vi "test - FGV Register and Unregister.vi"(8 "error in (no error)":errorcluster, 11 "TestCase in":refnum<class "testcase-Broadcast Registry.lvclass">) -> (0 "error out":errorcluster, 3 "TestCase out":refnum<class "testcase-Broadcast Registry.lvclass">)   [LabVIEW 2017, in "testcase-Broadcast Registry.lvclass"]
uses:
  testcase-Broadcast Registry.lvclass
  <vilib>/addons/_JKI Toolkits/VI Tester/TestCase.llb/TestCase.lvclass
  C:/Program Files (x86)/National Instruments/LabVIEW 2017/vi.lib/addons/_JKI Toolkits/VI Tester/TestCase.llb/TestCase.lvclass
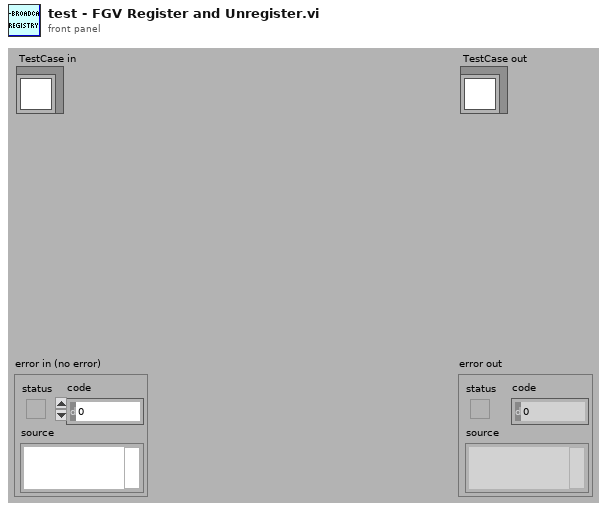
[diagram p1: front panel]
types:
  T1 = cluster{"response message":string[], "response message":string[], "response message":string[], "response message":string[], "response message":string[]}
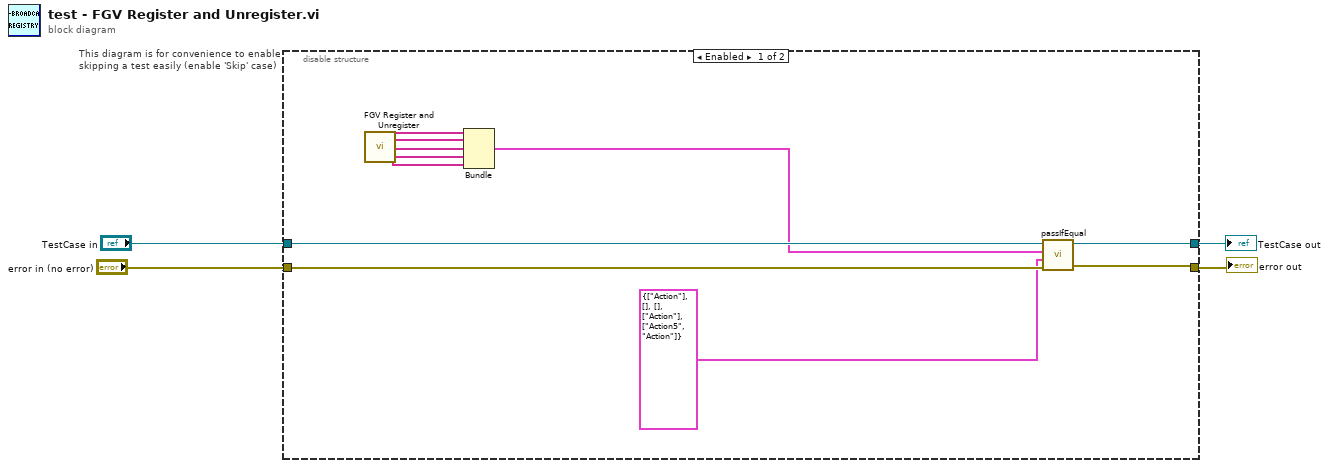
[diagram p0: block diagram]
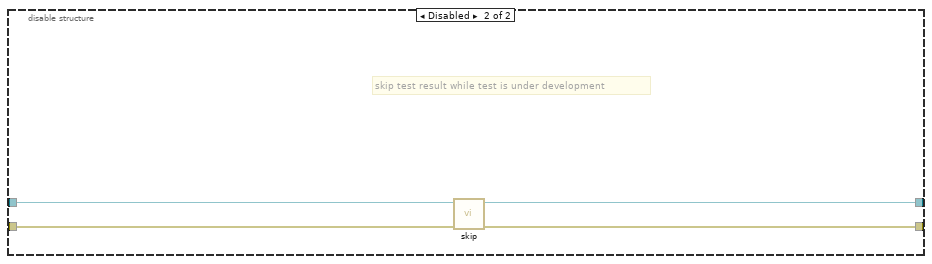
[diagram p2: hidden frame]
diagram:
  n1 = disable-structure "This diagram is for convenience to enable skipping a test easily (enable 'Skip' case)" shown="Enabled" {
    disable-tunnel: "TestCase in" -> [w13 w19]
    disable-tunnel: [w15 w17] -> w1
    disable-tunnel: [w14 w18] -> w3
    disable-tunnel: "error in (no error)" -> [w12 w16]
    frame Enabled {
      n2 = call "FGV Register and Unregister.vi"() -> (4:"response message"=w11:string[], 6:"response message"=w10:string[], 8:"response message"=w9:string[], 10:"response message"=w8:string[], 15:"response message"=w7:string[])  [unwired: 11 in]
      n3 = Bundle("response message"=w11, "response message"=w10, "response message"=w9, "response message"=w8, "response message"=w7) -> (w6:T1)  [unwired: 1 in]
      n4 = call-dynamic "passIfEqual.vi"("error in (no error)"=w12, "y"=T1 {"response message"=["Action"], "response message"=[], "response message"=[], "response message"=["Action"], "response message"=["Action5", "Action"]} ("output cluster"), "x"=w6, "TestCase in"=w13) -> ("error out"=w14:errorcluster, "TestCase out"=w15:refnum<class "testcase-Broadcast Registry.lvclass">)  [unwired: 6 in]
    }
    frame Disabled {
      # "skip test result while test is under development"
      n5 = call <vilib>:"skip.vi"("error in (no error)"=w16, "TestCase in"=w19) -> ("error out"=w18:errorcluster, "TestCase out"=w17:refnum<class "testcase-Broadcast Registry.lvclass">)  [unwired: 8 in]
    }
  }
  "error out" <- w3
  "TestCase out" <- w1
